vi "Directional Speed Sensors Page - Multi FPGA.vi"(8 "error in (no error)":errorcluster, 11 "Node Ptr":T1 format="%.0x") -> (0 "error out":errorcluster)   [LabVIEW 2015, in "Engine Simulation Toolkit System Explorer.lvlib"]
uses:
  Engine Simulation Toolkit System Explorer.lvlib
  <vilib>/NI Veristand/Custom Device API/Custom Device Item Ref.ctl
  Shared/Properties.vi
  <vilib>/NI Veristand/Custom Device API/Get Item Property (String Array).vi
  Shared/Constants and GUIDs.vi
  <vilib>/NI Veristand/Custom Device API/Custom Device API.lvlib
  Shared/Engine Simulation Toolkit Shared.lvlib
  <vilib>/NI Veristand/Custom Device Tools/Custom Device Utility Library/Custom Device Utility Library.lvlib
panel:
  in  "remove":bool
  in  "add":bool
  in  "DirSpeed listbox":i32[](listbox) caption="Available Directional Speed Sensors"
  in  "Header":cluster{"Section Name":string}={"Section Name"="Directional Speed Sensors"}
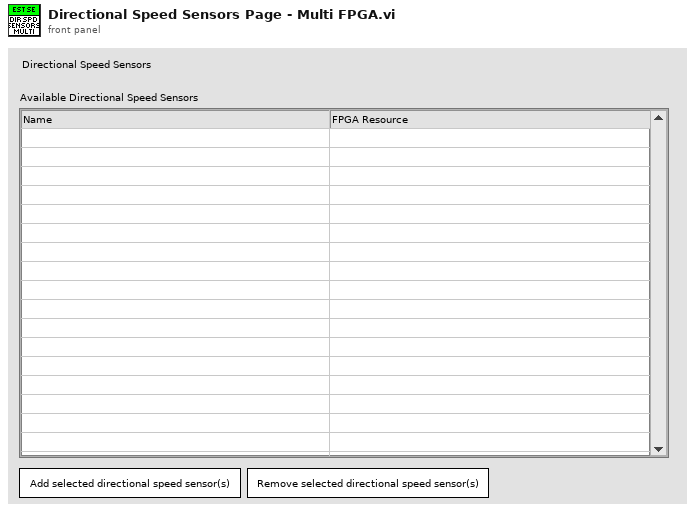
[diagram p1: front panel]
types:
  T1 = typedef "Custom Device API.lvlib/Custom Device Item Ref.ctl" = u64
  T2 = enum8{"Enabled", "Disabled", "Disabled and Grayed Out"}
  T3 = cluster{"ip list property name":string, string[]}[]
  T4 = typedef "Custom Device API.lvlib/Custom Device Commands.ctl" = enum16{"Default", "Item renamed", "Shutdown", "Dynamic button pressed"}
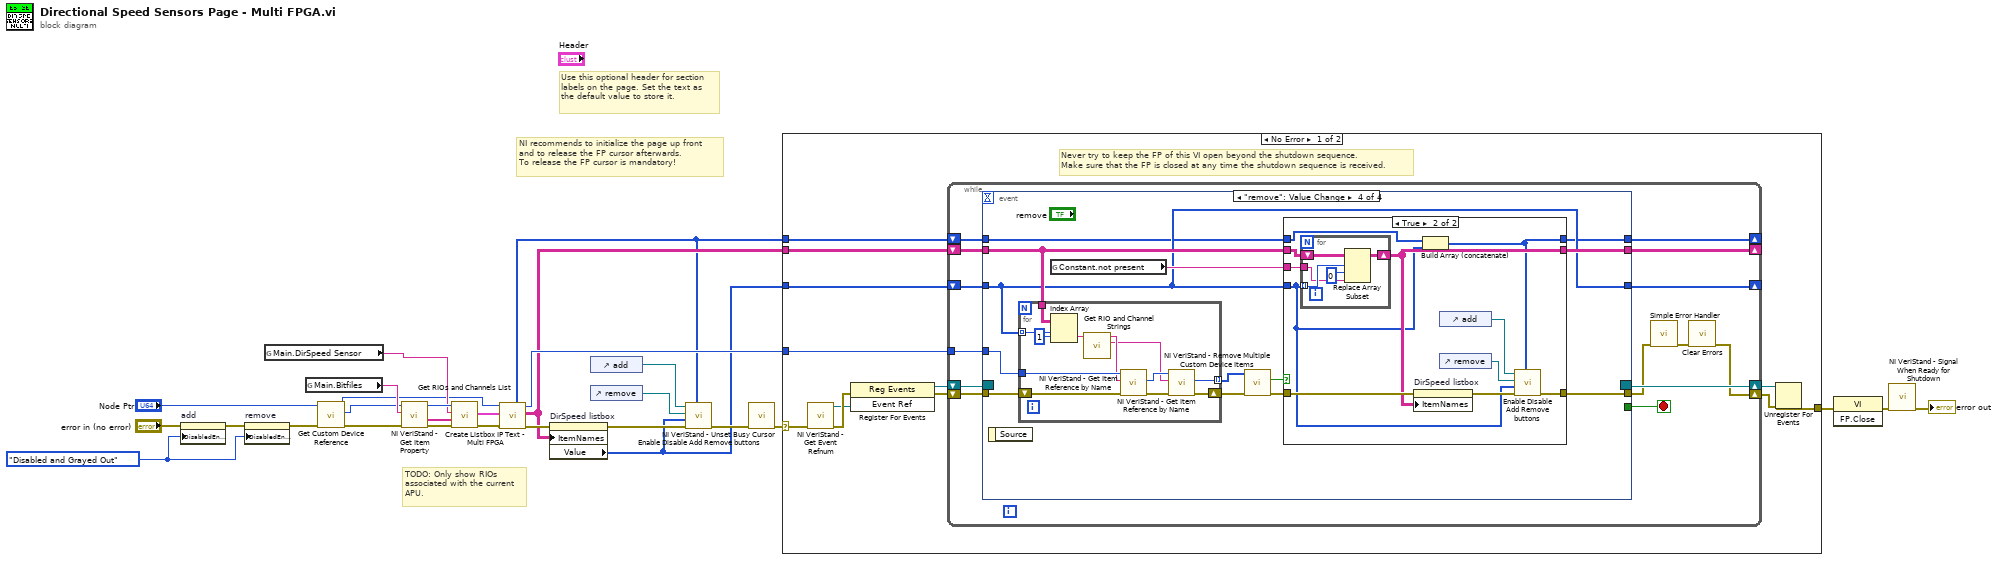
[diagram p0: block diagram]
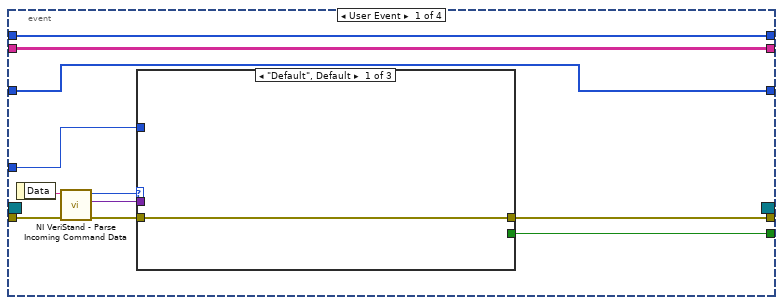
[diagram p2: hidden frame]
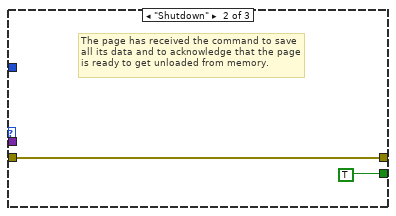
[diagram p3: hidden frame]
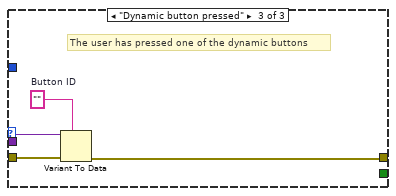
[diagram p4: hidden frame]
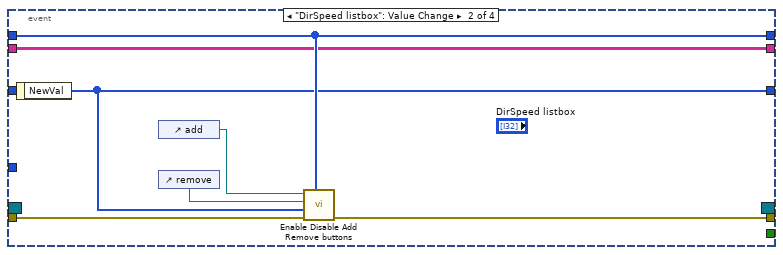
[diagram p5: hidden frame]
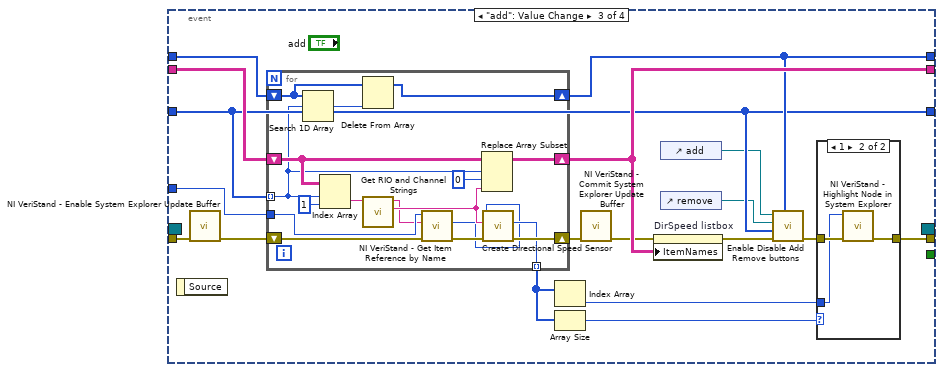
[diagram p6: hidden frame]
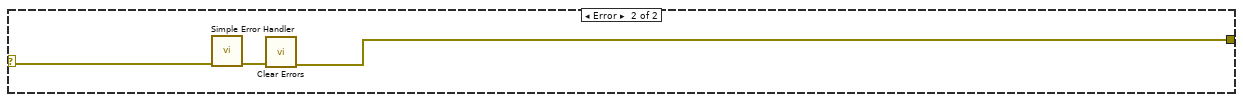
[diagram p9: hidden frame]
diagram:
  w19 = T2."Disabled and Grayed Out" ("Disabled")
  # "TODO: Only show RIOs\nassociated with the current\nAPU."
  # "Use this optional header for section labels on the page. Set the text as the default value to store it."
  # "NI recommends to initialize the page up front\nand to release the FP cursor afterwards.\nTo release the FP cursor is mandatory!"
  n1 = property on="add" class="Bool"(error in="error in (no error)", "DisabledEnum"=w19) -> (error out=w20:errorcluster)  [unwired: 1 in, 1 out]
  n2 = property on="remove" class="Bool"(error in=w20, "DisabledEnum"=w19) -> (error out=w12:errorcluster)  [unwired: 1 in, 1 out]
  n3 = global read "Properties.vi" "Main.DirSpeed Sensor"() -> (w4:string)
  n4 = global read "Properties.vi" "Main.Bitfiles"() -> (w7:string)
  n5 = call "Get Custom Device Reference.vi"("error in (no error)"=w12, "Item Ref in"="Node Ptr") -> ("error out"=w6:errorcluster, "Custom Device Ref"=w5:T1, "Item Ref out"=w1:T1)  [unwired: 7 in]
  n6 = call-poly <vilib>:"NI VeriStand - Get Item Property.vi"("error in (no error)"=w6, "Property Name"=w7, "Item Ref in"=w5) -> ("error out"=w10:errorcluster, "Value"=w8:string[], "Item Ref out"=w9:T1)  [unwired: 5 in, 1 out]
  n7 = call "Get RIOs and Channels List.vi"("error in (no error)"=w10, "rio names"=w8, "ip list property name"=w4, "Item Ref in"=w9) -> ("error out"=w3:errorcluster, "rios and channels"=w2:T3)  [unwired: 5 in, 1 out]
  n8 = call "Create Listbox IP Text - Multi FPGA.vi"("error in (no error)"=w3, "rios and analog replays"=w2, "Section Ref in"=w1) -> ("error out"=w22:errorcluster, "listbox text"=w21:string[][], "Section Ref out"=w23:T1, "not present item indexes"=w14:i32[])  [unwired: 5 in]
  n9 = property on="DirSpeed listbox" class="MCListbox (strict)"(error in=w22, "ItemNames"=w21) -> (error out=w16:errorcluster, "Value"=w13:i32[])  [unwired: 1 in, 1 out]
  n10 = control-ref of="add"() -> (w17:refnum<vi>)
  n11 = control-ref of="remove"() -> (w18:refnum<vi>)
  n12 = call "Enable Disable Add Remove buttons.vi"("not present item indexes"=w14, "error in (no error)"=w16, "selected items"=w13, "remove button"=w18, "add button"=w17) -> ("error out"=w15:errorcluster)  [unwired: 6 in]
  n13 = call <vilib>:"NI VeriStand - Unset Busy Cursor.vi"("error in (no error)"=w15) -> ("error out"=w25:errorcluster)  [unwired: 10 out]
  n14 = case shown="No Error" w25 {
    selector: w25 -> [w32 w165]
    tunnel: [w37 w163] -> w28
    tunnel: w23 -> [w33 _]
    tunnel: w21 -> [w31 _]
    tunnel: w14 -> [w30 _]
    tunnel: w13 -> [w29 _]
    frame No Error {
      # "Never try to keep the FP of this VI open beyond the shutdown sequence.\nMake sure that the FP is closed at any time the shutdown sequence is received."
      n15 = call <vilib>:"NI VeriStand - Get Event Refnum.vi"("error in (no error)"=w32) -> ("error out"=w40:errorcluster, "Event Ref"=w36:refnum<user-event>)  [unwired: 9 out]
      n16 = register-events(error in=w40, w36) -> (reference out=w34:refnum<event-registration>, error out=w35:errorcluster)  [unwired: 1 in]
      n17 = while {
        tunnel: w33 -> [w50]
        shift-right: [w47] -> w38
        shift-left: w35 -> [w53]
        shift-right: [w54] -> w39
        shift-left: w34 -> [w52]
        shift-right: [w44] -> _
        shift-left: w29 -> [w43]
        shift-right: [w41] -> _
        shift-left: w30 -> [w45]
        shift-right: [w42] -> _
        shift-left: w31 -> [w46]
        stop <- w51 stop-if-true
        n18 = event shown="[3] \"remove\": Value Change" {
          selector: w52 -> [_ _ _ _]
          dyn-events: [_ _ _ _] -> w54
          timeout: _ -> [_ _ _ _]
          tunnel: w53 -> [w65 w79 w97 w130]
          tunnel: [w61 _ _ _] -> w51
          tunnel: [w60 w78 w82 w131] -> w49
          tunnel: w50 -> [w59 _ w96 w129]
          tunnel: w46 -> [w56 w73 w95 w124]
          tunnel: w45 -> [w55 w75 w94 w120]
          tunnel: [w57 w74 w89 w121] -> w44
          tunnel: w43 -> [w57 _ w89 w121]
          tunnel: [w56 w73 w92 w122] -> w42
          tunnel: [w55 w75 w90 w119] -> w41
          event User Event {
            n19 = event-data() -> ("Data"=w64:string)  [unwired: 1 out]
            n20 = call <vilib>:"NI VeriStand - Parse Incoming Command Data.vi"("error in (no error)"=w65, "Incoming data"=w64) -> ("error out"=w63:errorcluster, "Outgoing data"=w58:variant, "Action"=w62:T4)  [unwired: 7 out]
            n21 = case shown="\"Default\", Default" w62 {
              tunnel: w63 -> [w66 w67 w72]
              tunnel: [_ TRUE _] -> w61
              tunnel: [w66 w67 w69] -> w60
              tunnel: w59 -> [_ _ _]
              tunnel: w58 -> [_ _ w71]
              frame "Default", Default {
              }
              frame "Shutdown" {
                # "The page has received the command to save all its data and to acknowledge that the page is ready to get unloaded from memory."
              }
              frame "Dynamic button pressed" {
                w70 = ""  # Button ID
                # "The user has pressed one of the dynamic buttons"
                n22 = Variant To Data(error in=w72, type=w70, Variant=w71) -> (error out=w69:errorcluster)  [unwired: 1 out]
              }
            }
          }
          event "DirSpeed listbox": Value Change {
            n23 = event-data() -> ("NewVal"=w74:i32[])  [unwired: 1 out]
            n24 = control-ref of="add"() -> (w77:refnum<vi>)
            n25 = control-ref of="remove"() -> (w76:refnum<vi>)
            n26 = call "Enable Disable Add Remove buttons.vi"("not present item indexes"=w75, "error in (no error)"=w79, "selected items"=w74, "remove button"=w76, "add button"=w77) -> ("error out"=w78:errorcluster)  [unwired: 6 in]
          }
          event "add": Value Change {
            n27 = event-data() -> ()  [unwired: 2 out]
            n28 = call <vilib>:"NI VeriStand - Enable System Explorer Update Buffer.vi"("error in (no error)"=w97) -> ("error out"=w85:errorcluster)  [unwired: 10 in]
            n29 = for {
              tunnel: w96 -> [w104]
              shift-right: [w118] -> w93
              shift-left: w85 -> [w106]
              tunnel: w89 -> [w113] mode=indexing
              shift-right: [w115] -> w92
              shift-left: w95 -> [w116]
              shift-right: [w110] -> w90
              shift-left: w94 -> [w112]
              tunnel: [w109] -> w84 mode=indexing
              n30 = Search 1D Array(1D array=w112, element=w113) -> (index of element=w111:i32)  [unwired: 1 in]
              n31 = Index Array(array=w116, index (row)=w113, index (col)=1 ("disabled index (col)")) -> (element=w108:string)
              n32 = Delete From Array(array=w112, index=w111) -> (array with subset deleted=w110:i32[])  [unwired: 1 in, 1 out]
              n33 = call "Get RIO and Channel Strings.vi"("rio/channel"=w108) -> ("channel"=w107:string, "rio"=w102:string)  [unwired: 9 in]
              n34 = call <vilib>:"NI VeriStand - Get Item Reference by Name.vi"("error in (no error)"=w106, "Item Name"=w102, "Parent Ref in"=w104) -> ("error out"=w105:errorcluster, "Item Ref"=w103:T1)  [unwired: 5 in, 2 out]
              n35 = Replace Array Subset(array=w116, new element=w107, index (row)=w113, index (col)=0 ("disabled index (col)")) -> (w115:string[][])
              n36 = call "Create Directional Speed Sensor.vi"("error in (no error)"=w105, "dir speed sensor name"=w107, "Section Ptr"=w103) -> ("error out"=w118:errorcluster, "dir speed sensor ref"=w109:T1)  [unwired: 6 in, 1 out]
            }
            n37 = Index Array(array=w84) -> (element=w80:T1)  [unwired: 1 in]
            n38 = Array Size(array=w84) -> (size(s)=w83:i32)
            n39 = call <vilib>:"NI VeriStand - Commit System Explorer Update Buffer.vi"("error in (no error)"=w93) -> ("error out"=w86:errorcluster)  [unwired: 10 in]
            n40 = property on="DirSpeed listbox" class="MCListbox (strict)"(error in=w86, "ItemNames"=w92) -> (error out=w91:errorcluster)  [unwired: 1 in, 1 out]
            n41 = control-ref of="add"() -> (w88:refnum<vi>)
            n42 = control-ref of="remove"() -> (w87:refnum<vi>)
            n43 = call "Enable Disable Add Remove buttons.vi"("not present item indexes"=w90, "error in (no error)"=w91, "selected items"=w89, "remove button"=w87, "add button"=w88) -> ("error out"=w81:errorcluster)  [unwired: 6 in]
            n44 = case shown="1" w83 {
              tunnel: [w98 w100] -> w82
              tunnel: w81 -> [w98 w101]
              tunnel: w80 -> [_ w99]
              frame Default {
              }
              frame 1 {
                n45 = call <vilib>:"NI VeriStand - Highlight Node in System Explorer.vi"("error in (no error)"=w101, "Item Ref in"=w99) -> ("error out"=w100:errorcluster)  [unwired: 8 in, 1 out]
              }
            }
          }
          event "remove": Value Change {
            n46 = event-data() -> ()  [unwired: 2 out]
            n47 = for {
              tunnel: w121 -> [w161] mode=indexing
              tunnel: w124 -> [w162]
              tunnel: w129 -> [w158]
              tunnel: [w157] -> w127 mode=indexing
              shift-right: [w155] -> w128
              shift-left: w130 -> [w159]
              n48 = Index Array(array=w162, index (row)=w161, index (col)=1 ("disabled index (col)")) -> (element=w153:string)
              n49 = call "Get RIO and Channel Strings.vi"("rio/channel"=w153) -> ("channel"=w151:string, "rio"=w152:string)  [unwired: 9 in]
              n50 = call <vilib>:"NI VeriStand - Get Item Reference by Name.vi"("error in (no error)"=w159, "Item Name"=w152, "Parent Ref in"=w158) -> ("error out"=w156:errorcluster, "Item Ref"=w154:T1)  [unwired: 5 in, 2 out]
              n51 = call <vilib>:"NI VeriStand - Get Item Reference by Name.vi"("error in (no error)"=w156, "Item Name"=w151, "Parent Ref in"=w154) -> ("error out"=w155:errorcluster, "Item Ref"=w157:T1)  [unwired: 5 in, 2 out]
            }
            n52 = global read "Constants and GUIDs.vi" "Constant.not present"() -> (w123:string)
            n53 = call <vilib>:"NI VeriStand - Remove Multiple Custom Device Items.vi"("error in (no error)"=w128, "Item Refs in"=w127) -> ("error out"=w126:errorcluster, "Deleted?"=w125:bool)  [unwired: 8 in]
            n54 = case shown="True" w125 {
              tunnel: [w133 w144] -> w131
              tunnel: w126 -> [w133 w141]
              tunnel: w121 -> [_ w136]
              tunnel: w124 -> [w134 w140]
              tunnel: w123 -> [_ w139]
              tunnel: [w134 w138] -> w122
              tunnel: w120 -> [w132 w137]
              tunnel: [w132 w135] -> w119
              frame False {
              }
              frame True {
                n55 = for {
                  tunnel: w136 -> [w148] mode=indexing
                  shift-right: [w149] -> w138
                  shift-left: w140 -> [w150]
                  tunnel: w139 -> [w146]
                  n56 = Replace Array Subset(array=w150, new element=w146, index (row)=w148, index (col)=0 ("disabled index (col)")) -> (w149:string[][])
                }
                n57 = property on="DirSpeed listbox" class="MCListbox (strict)"(error in=w141, "ItemNames"=w138) -> (error out=w145:errorcluster)  [unwired: 1 in, 1 out]
                n58 = Build Array (concatenate)(w137, w136) -> (w135:i32[])
                n59 = control-ref of="add"() -> (w143:refnum<vi>)
                n60 = control-ref of="remove"() -> (w142:refnum<vi>)
                n61 = call "Enable Disable Add Remove buttons.vi"("not present item indexes"=w135, "error in (no error)"=w145, "selected items"=w136, "remove button"=w142, "add button"=w143) -> ("error out"=w144:errorcluster)  [unwired: 6 in]
              }
            }
          }
        }
        n62 = call <vilib>:"Simple Error Handler.vi"("error in (no error)"=w49) -> ("error out"=w48:errorcluster)  [unwired: 1 in, 7 out]
        n63 = call <vilib>:"Clear Errors.vi"("error in (no error)"=w48) -> ("error out"=w47:errorcluster)  [unwired: 1 in, 5 out]
      }
      n64 = Unregister For Events(event registration refnum=w39, error in=w38) -> (error out=w37:errorcluster)
    }
    frame Error {
      n65 = call <vilib>:"Simple Error Handler.vi"("error in (no error)"=w165) -> ("error out"=w164:errorcluster)  [unwired: 1 in, 7 out]
      n66 = call <vilib>:"Clear Errors.vi"("error in (no error)"=w164) -> ("error out"=w163:errorcluster)  [unwired: 1 in, 5 out]
    }
  }
  n67 = invoke class="VI" method="FP.Close"(error in=w28) -> (error out=w27:errorcluster)  [unwired: 2 in, 2 out]
  n68 = call <vilib>:"NI VeriStand - Signal When Ready for Shutdown.vi"("error in (no error)"=w27) -> ("error out"=→"error out":errorcluster)  [unwired: 10 out]
